vi "New Minor Frame.vi"(8 "error in":errorcluster, 9 "frameTime uS (200)":i32=200, 10 "Scheduled Message Config in":T1[](array[typedef]), 11 "name":string) -> (0 "error out":errorcluster, 3 "new minor frame":refnum<k24>)   [LabVIEW 2020, in "Ballard_1553_Hardware_ni.lvlib"]
uses:
  Ballard_1553_Hardware_ni.lvlib
  C:/Users/Administrator/Desktop/GIT/Ballard-MIL-STD-1553-Custom-Device/Source/System Explorer/SubVIs/Parse XML Ballard/1.2/BTIXML_SerDes.dll
  Ballard-MIL-STD-1553-Custom-Device/Source/System Explorer/SubVIs/Parse XML Ballard/1.2/BTIXML_SerDes.dll
  _typedefs/schedItem1553_type.ctl
  _typedefs/frame_entry_type.ctl
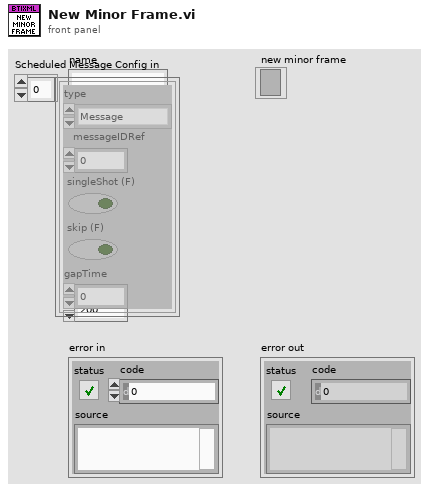
[diagram p1: front panel]
types:
  T1 = typedef "Ballard_1553_Hardware_ni.lvlib/schedItem1553_type.ctl" = cluster{"type":T2, "messageIDRef":i32, "singleShot (F)":bool, "skip (F)":bool, "gapTime":dbl}
  T2 = typedef "Ballard_1553_Hardware_ni.lvlib/frame_entry_type.ctl" = enum16{"Message", "Gap", "Pulse", "Log", "Pause", "Restart", "Halt"}
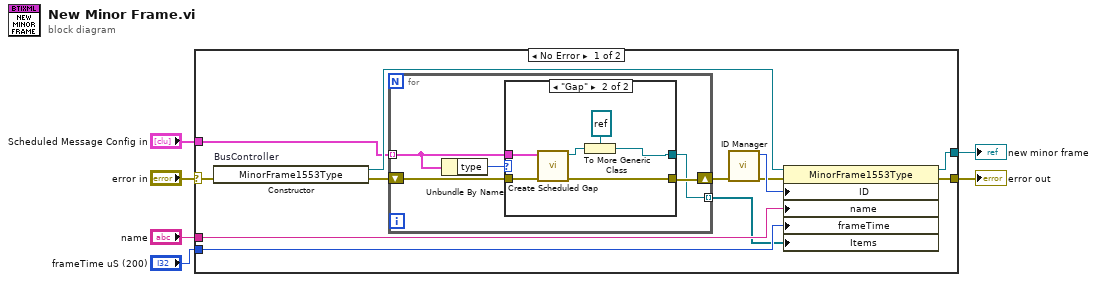
[diagram p0: block diagram]
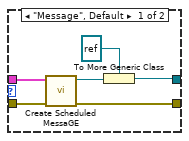
[diagram p2: hidden frame]
diagram:
  n1 = case shown="No Error" "error in" {
    selector: "error in" -> [w18 w36]
    tunnel: [w17 w36] -> w5
    tunnel: [w16 _] -> w2
    tunnel: "name" -> [w12 _]
    tunnel: "Scheduled Message Config in" -> [w10 _]
    tunnel: "frameTime uS (200)" -> [w11 _]
    frame No Error {
      n2 = constructor on="BusController" class="MinorFrame1553Type"(error in=w18) -> (reference out=w15:refnum<k24>, error out=w9:errorcluster)  [unwired: 2 in, 1 out]
      n3 = for {
        tunnel: w10 -> [w20] mode=indexing
        shift-right: [w22] -> w7
        shift-left: w9 -> [w23]
        tunnel: [w21] -> w8 mode=indexing
        n4 = Unbundle By Name(w20) -> ("type"=w19:T2)
        n5 = case shown="\"Gap\"" w19 {
          tunnel: w20 -> [w29 w34]
          tunnel: w23 -> [w28 w35]
          tunnel: [w27 w30] -> w22
          tunnel: [w24 w31] -> w21
          frame "Message", Default {
            n6 = call "Create Scheduled MessaGE.vi"("error in"=w28, "1553 Scheduled Message Configuration in"=w29) -> ("error out"=w27:errorcluster, "message out"=w25:refnum<k24>)  [unwired: 8 in]
            n7 = To More Generic Class(target class=refnum<k24> refnum, reference=w25) -> (generic class reference=w24:refnum<k24>)
          }
          frame "Gap" {
            n8 = call "Create Scheduled Gap.vi"("error in"=w35, "1553 Scheduled Message Configuration in"=w34) -> ("error out"=w30:errorcluster, "gap item out"=w33:refnum<k24>)  [unwired: 8 in]
            n9 = To More Generic Class(target class=refnum<k24> refnum, reference=w33) -> (generic class reference=w31:refnum<k24>)
          }
        }
      }
      n10 = call "ID Manager.vi"("error in"=w7) -> ("error out"=w13:errorcluster, "ID out"=w14:i32)  [unwired: 9 in]
      n11 = property class="MinorFrame1553Type"(reference=w15, error in=w13, "ID"=w14, "name"=w12, "frameTime"=w11, "Items"=w8) -> (reference out=w16:refnum<k24>, error out=w17:errorcluster)
    }
    frame Error {
    }
  }
  "error out" <- w5
  "new minor frame" <- w2
